vi "Set Frequency.vi"(0 "reference":refnum<k15>, 5 "Frequency (Hz)":dbl, 11 "error in (no error)":errorcluster) -> (4 "reference out":refnum<k15>, 15 "error out":errorcluster)   [LabVIEW 2023, in "NI-568x RF Power Meter.lvlib" / "SG 2250 Path Accessor.lvclass"]
uses:
  SG 2250 Path Accessor.lvclass
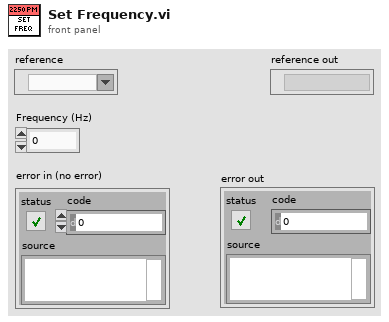
[diagram p1: front panel]
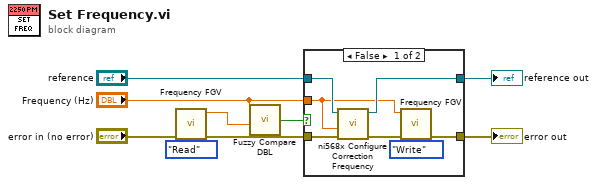
[diagram p0: block diagram]
diagram:
  n1 = call "Frequency FGV.vi"("Action"=enum16{"Write", "Read"}."Read", "error in (no error)"="error in (no error)") -> ("error out"=w6:errorcluster, "Frequency (Hz)"=w5:dbl)  [unwired: 5 in]
  n2 = call "Fuzzy Compare DBL.vi"("A"="Frequency (Hz)", "B"=w5) -> ("Fuzzy Equal?"=w7:bool)  [unwired: 5 in]
  n3 = case shown="False" w7 {
    tunnel: w6 -> [w11 w18]
    tunnel: "Frequency (Hz)" -> [w10 _]
    tunnel: "reference" -> [w14 w17]
    tunnel: [w16 w18] -> w3
    tunnel: [w13 w17] -> w2
    frame False {
      n4 = call <instrlib>:"ni568x Configure Correction Frequency.vi"("error in"=w11, "frequency"=w10, "instrument handle"=w14) -> ("error out"=w12:errorcluster, "instrument handle out"=w13:refnum<k15>)  [unwired: 7 in]
      n5 = call "Frequency FGV.vi"("Action"=enum16{"Write", "Read"}."Write", "error in (no error)"=w12, "Write Value (Hz)"=w10) -> ("error out"=w16:errorcluster)  [unwired: 4 in, 1 out]
    }
    frame True {
    }
  }
  "error out" <- w3
  "reference out" <- w2
